vi "DSF.Engine.Framework.Process Rx.vi"(8 "error in (no error)":errorcluster, 11 "Framework in":refnum<class "Framework.lvclass">) -> (0 "error out":errorcluster, 3 "Framework out":refnum<class "Framework.lvclass">)   [LabVIEW 2016, in "DSF.Engine.lvlib" / "Framework.lvclass"]
uses:
  Framework.lvclass
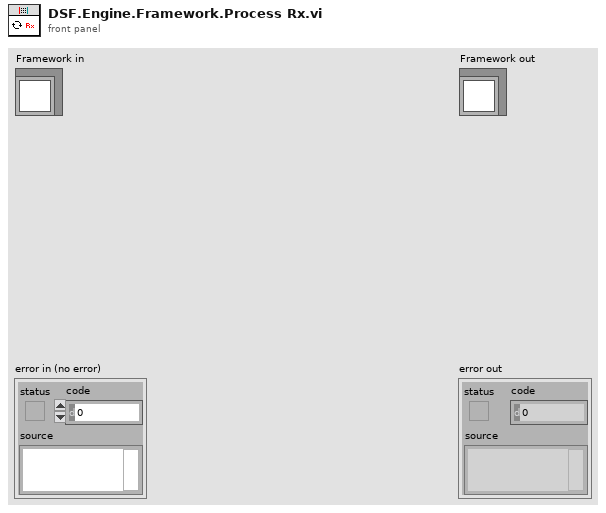
[diagram p1: front panel]
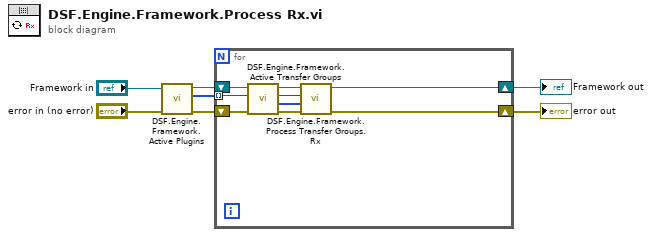
[diagram p0: block diagram]
diagram:
  n1 = call "DSF.Engine.Framework.Active Plugins.vi"("error in (no error)"="error in (no error)", "Framework in"="Framework in") -> ("error out"=w3:errorcluster, "active Plugin indices"=w5:i32[], "Framework out"=w6:refnum<class "Framework.lvclass">)  [unwired: 7 in]
  n2 = for {
    shift-right: [w11] -> w1
    shift-left: w6 -> [w16]
    tunnel: w5 -> [w10] mode=indexing
    shift-right: [w12] -> w2
    shift-left: w3 -> [w15]
    n3 = call "DSF.Engine.Framework.Active Transfer Groups.vi"("error in (no error)"=w15, "Plugin index in"=w10, "Framework in"=w16) -> ("error out"=w13:errorcluster, "active Transfer Group indicies"=w9:i32[], "Plugin index out"=w8:i32, "Framework out"=w14:refnum<class "Framework.lvclass">)  [unwired: 5 in]
    n4 = call "DSF.Engine.Framework.Process Transfer Groups.Rx.vi"("error in (no error)"=w13, "Transfer Group indicies"=w9, "Plugin index"=w8, "Framework in"=w14) -> ("error out"=w12:errorcluster, "Framework out"=w11:refnum<class "Framework.lvclass">)  [unwired: 6 in]
  }
  "error out" <- w2
  "Framework out" <- w1
